vi "Do.vi"(8 "error in (no error)":errorcluster, 10 "Actor in":refnum<class "Actor.lvclass">, 11 "Configure Data Marker [DM] Msg":refnum<class "Configure Data Marker [DM] Msg.lvclass">) -> (0 "error out":errorcluster, 2 "Actor out":refnum<class "Actor.lvclass">)   [LabVIEW 2015, in "CS++Fgen.lvlib" / "Configure Data Marker [DM] Msg.lvclass"]
doc: "This VI delivers the message to the actor by calling the appropriate method(s) on the actor."
uses:
  Configure Data Marker [DM] Msg.lvclass
  <vilib>/ActorFramework/Actor/Actor.lvclass
  CS++Fgen/CS++Fgen.lvclass
  CSPP_Core/Actors/CS++PVMonitor Messages/CS++PVUpdate Msg/CS++PVUpdate Msg.lvclass/CS++PVUpdate Msg.ctl
  CSPP_Core/Classes/CS++ProcessVariables/ProcessVariable/PV.lvclass/PV.ctl
  Configure Data Marker [DM] Msg.lvclass/Configure Data Marker [DM] Msg.ctl
  CSPP_Core/Classes/CS++ProcessVariables/ProcessVariable/PV.lvclass
  CSPP_Core/Actors/CS++PVMonitor Messages/CS++PVUpdate Msg/CS++PVUpdate Msg.lvclass
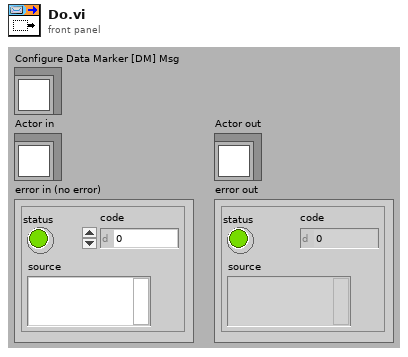
[diagram p1: front panel]
types:
  T1 = cluster{"Source Channel (\"\")":string, "Marker Name (\"\")":string, "Bit Position":i32, "Destination Terminal (None)":string}
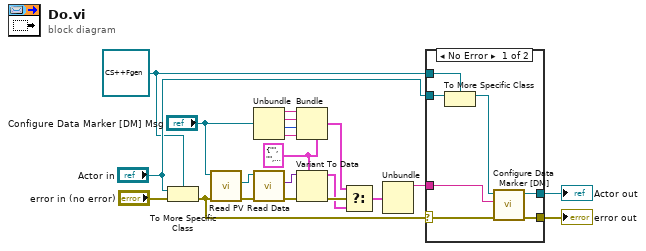
[diagram p0: block diagram]
diagram:
  w13 = T1 {"Source Channel (\"\")"="", "Marker Name (\"\")"="", "Bit Position"=0, "Destination Terminal (None)"=""} ("Type")
  w17 = refnum<class "CS++Fgen.lvclass"> refnum ("Actor in")
  n1 = To More Specific Class(target class=w17, reference="Actor in", error in="error in (no error)") -> (error out=w6:errorcluster)  [unwired: 1 out]
  n2 = call "Read PV.vi"("error in (no error)"=w6, "CS++PVUpdate Msg in"="Configure Data Marker [DM] Msg") -> ("error out"=w16:errorcluster, "PV"=w12:refnum<class "PV.lvclass">)  [unwired: 7 in, 1 out]
  n3 = Unbundle ("Pre-Unbundler")("Configure Data Marker [DM] Msg") -> (w4:string, w3:string, w2:i32, w1:string)
  n4 = call "Read Data.vi"("error in (no error)"=w16, "PV in"=w12) -> ("error out"=w10:errorcluster, "Data"=w11:variant)  [unwired: 7 in, 1 out]
  n5 = Bundle ("Pre-Bundler")(cluster=w13, "Source Channel (\"\")"=w4, "Marker Name (\"\")"=w3, "Bit Position"=w2, "Destination Terminal (None)"=w1) -> (w14:T1)
  n6 = Variant To Data(error in=w10, type=w13, Variant=w11) -> (data=w8:T1, error out=w15:errorcluster)
  n7 = Select ("MainSelect")(t=w14, s=w15, f=w8) -> (s? t:f=w9:T1)
  n8 = Unbundle ("Main-Unbundler")(w9) -> ("Source Channel (\"\")"=w5:string)  [unwired: 3 out]
  n9 = case shown="No Error" w6 {
    selector: w6 -> [w26 w30]
    tunnel: [w28 w30] -> w20
    tunnel: [w27 w29] -> w19
    tunnel: "Actor in" -> [w25 w29]
    tunnel: w17 -> [w24 _]
    tunnel: w5 -> [w22 _]
    frame No Error {
      n10 = To More Specific Class(target class=w24, reference=w25) -> (specific class reference=w23:refnum<class "CS++Fgen.lvclass">)  [unwired: 1 in, 1 out]
      n11 = call "Configure Data Marker [DM].vi"("error in (no error)"=w26, "Source Channel (\"\")"=w22, "CS++Fgen in"=w23) -> ("error out"=w28:errorcluster, "CS++Fgen out"=w27:refnum<class "CS++Fgen.lvclass">)  [unwired: 7 in]
    }
    frame Error {
    }
  }
  "error out" <- w20
  "Actor out" <- w19
